vi "ME_acquire_4.vi"() -> ()   [LabVIEW 2015]
doc: "Use this template to build a producer/consumer design pattern. Use this template when you need to execute a process, such as data analysis, when a data source, such as a triggered acquisition, produces data at an uneven rate and you need to execute the process when the data becomes available."
uses:
  Mode.ctl
  oxford_driver/Oxford Drivers/BUSGEN.LLB/OxfordAddress.ctl
  <vilib>/Utility/file.llb/Write Delimited Spreadsheet (DBL).vi
  <vilib>/express/express arith-compare/Formula/XNode/ExpressFormulaBlockNode.xnode
  <vilib>/gmath/NI_Gmath.lvlib
panel:
  out "Actual B Field (T)":dbl
  out "Actual Temperature (K)":dbl
  out "Actual Current (pA)":dbl
  in  "Sweep Field":bool
  in  "Tab Control":T1(tab)
  out "P(T)":cluster{dbl[], dbl[]}(graph)
  out "I(T)":cluster{dbl[], dbl[]}(graph)
  in  "Set temperature (K)":dbl=4.5
  in  "Temp Ramping Rate (K/min)":dbl=10.0
  in  "Heater Range":enum16{"Off", "Low", "Medium", "High"}(ring)
  in  "Heater On/Off":bool
  out "I(B) /Averaged/":cluster{"B array":dbl[], dbl[]}[](graph)
  out "I(B) 3":cluster{dbl[], dbl[]}[](graph)
  in  "Go to Set":bool
  in  "Set Field (T)":dbl=0.3
  in  "Field To Zero":bool
  in  "Sweep Rate (T/min)":dbl=2.0 format="%.6f"
  in  "Min Field (T)":dbl
  in  "Max Field (T)":dbl
  out "Up/Down":bool
  in  "IV converter":refnum<visa-resource-name>="GPIB0::20::INSTR"
  in  "Magnetic Field":refnum<visa-resource-name>="GPIB0::21::INSTR"
  out "Time Lag":dbl=0.0500025749206543
  in  "Lake Shore":refnum<visa-resource-name>="GPIB0::11::INSTR"
  in  "Temp Refresh (s)":dbl=1.0
  in  "Sampling rate (Hz)":dbl=20.0
  in  "Gain (V/A)":dbl=1000.0
  in  "Sample area (mm^2)":dbl
  in  "dt (s)":dbl=0.05
  in  "Temp/Magnetic Field":bool
  out "Save":dbl[][](array[numeric])
  out "output array":dbl[][](array[numeric])
  out "index":i8
  out "Read?":bool
  out "Magnetic Field (T)":dbl[](array[numeric])
  out "Reset":bool
  out "Measured Current (pA)":dbl[](array[numeric])
  out "Elapsed Time (s)":dbl[](array[numeric])
  out "Start time":timestamp
  in  "Enum":T2
  out "B array":dbl[](array[numeric])
  in  "dB (T)":dbl=0.0001
  in  "Counter":i8
  out "L magnet (H)":dbl
  out "R magnet (mOhm)":dbl
  out "Actual Current (R0)":dbl
  out "Actual Field (T)":dbl
  out "Temperature array":dbl[](array[numeric])
  in  "New Measurement File":bool
  out "Measurement File":path
  out "refnum out":refnum<file>
  in  "Measuring":bool
  in  "Measure (Start/Pause)":bool
  in  "stop":bool
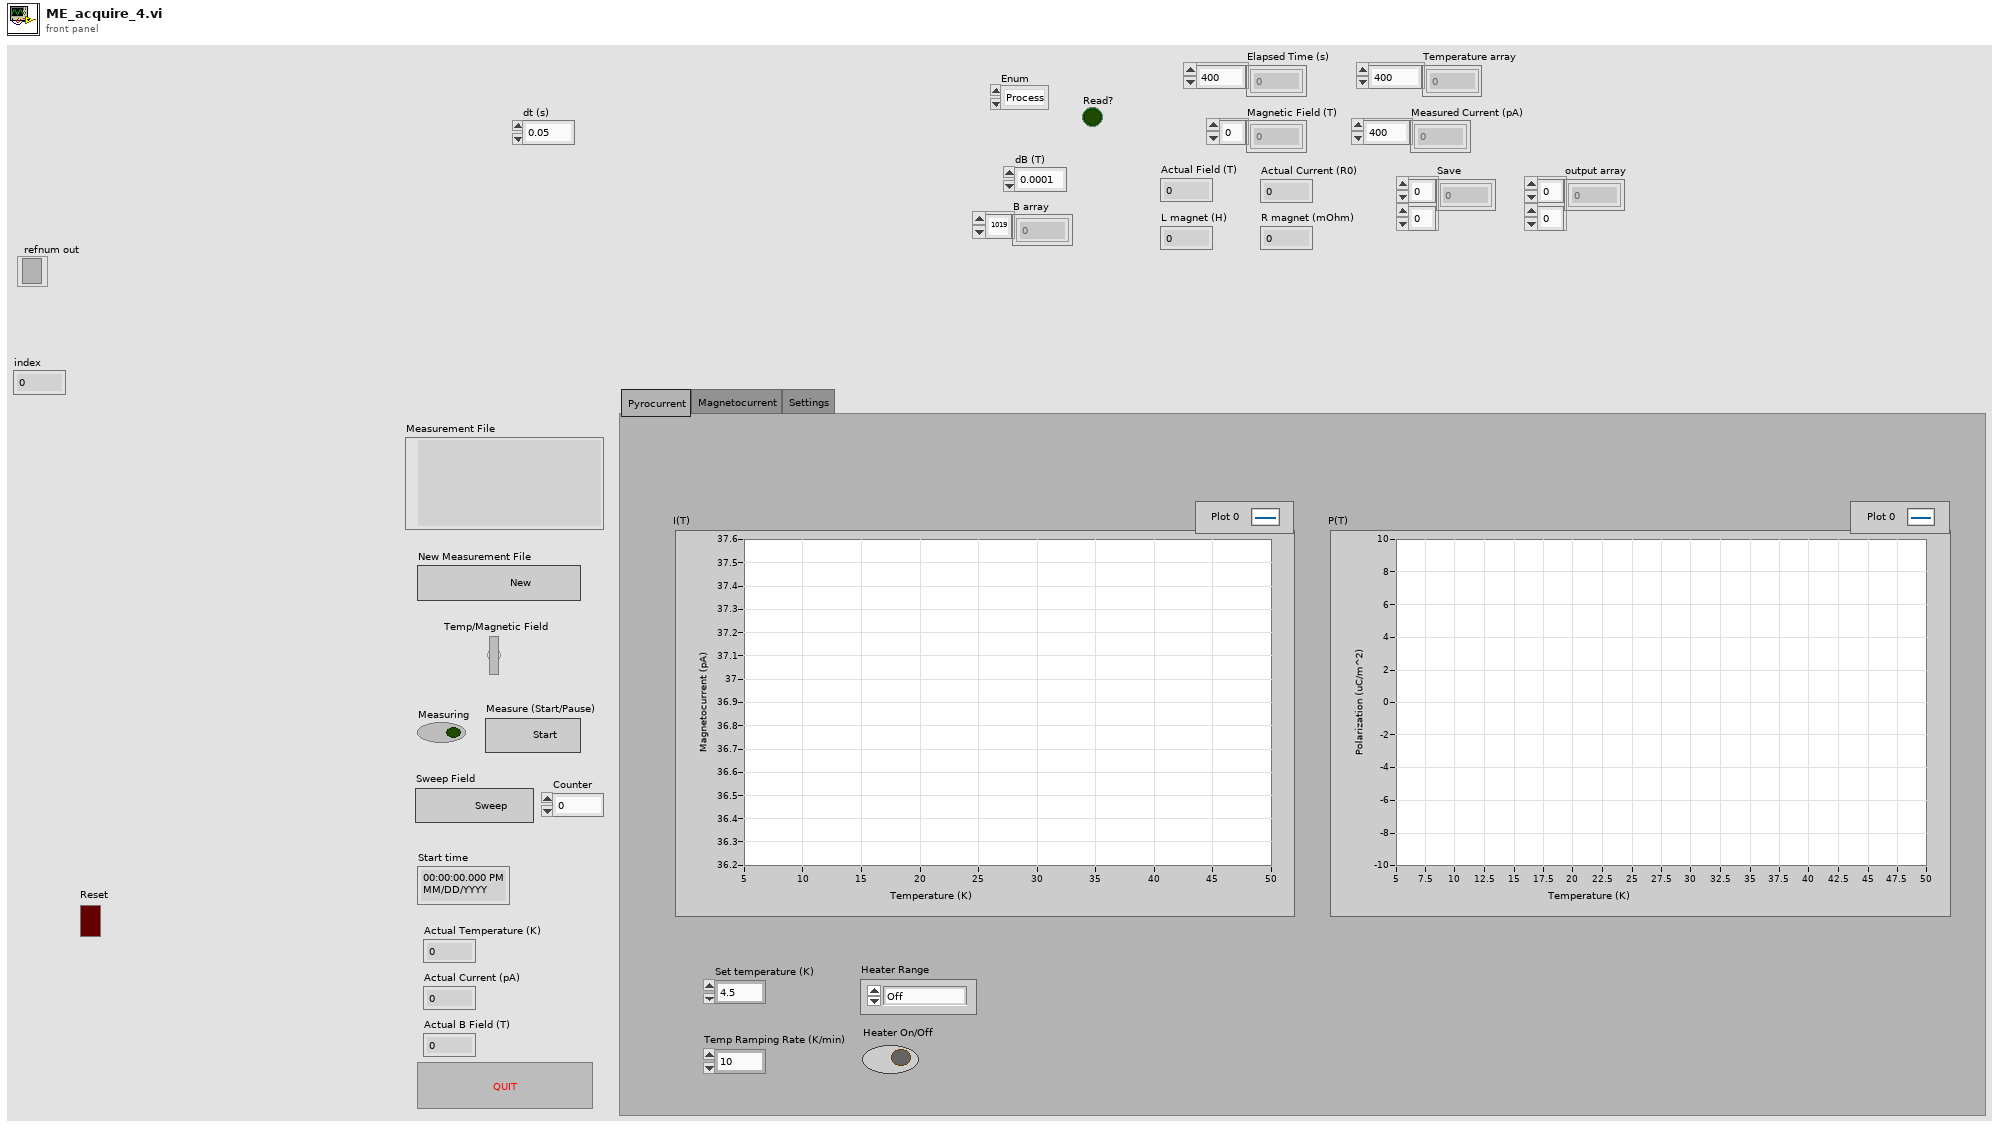
[diagram p1: front panel]
types:
  T1 = enum32{"Pyrocurrent", "Magnetocurrent", "Settings"}
  T2 = typedef "Mode.ctl" = enum16{"Process", "Plot", "Save", "Return"}
  T3 = enum16{"open", "replace", "create", "open or create", "replace or create", "replace or create with confirmation"}
  T4 = typedef "OxfordAddress.ctl" = cluster{"Com Port":i32, "ISOBUS Address":i32, "GPIB Address":i16, "Communication":enum16{"RS232", "ISOBUS", "GPIB", "Gateway"}}
  T5 = cluster{"seconds since 1Jan1904":timestamp, "read buffer":string, "read buffer":string}
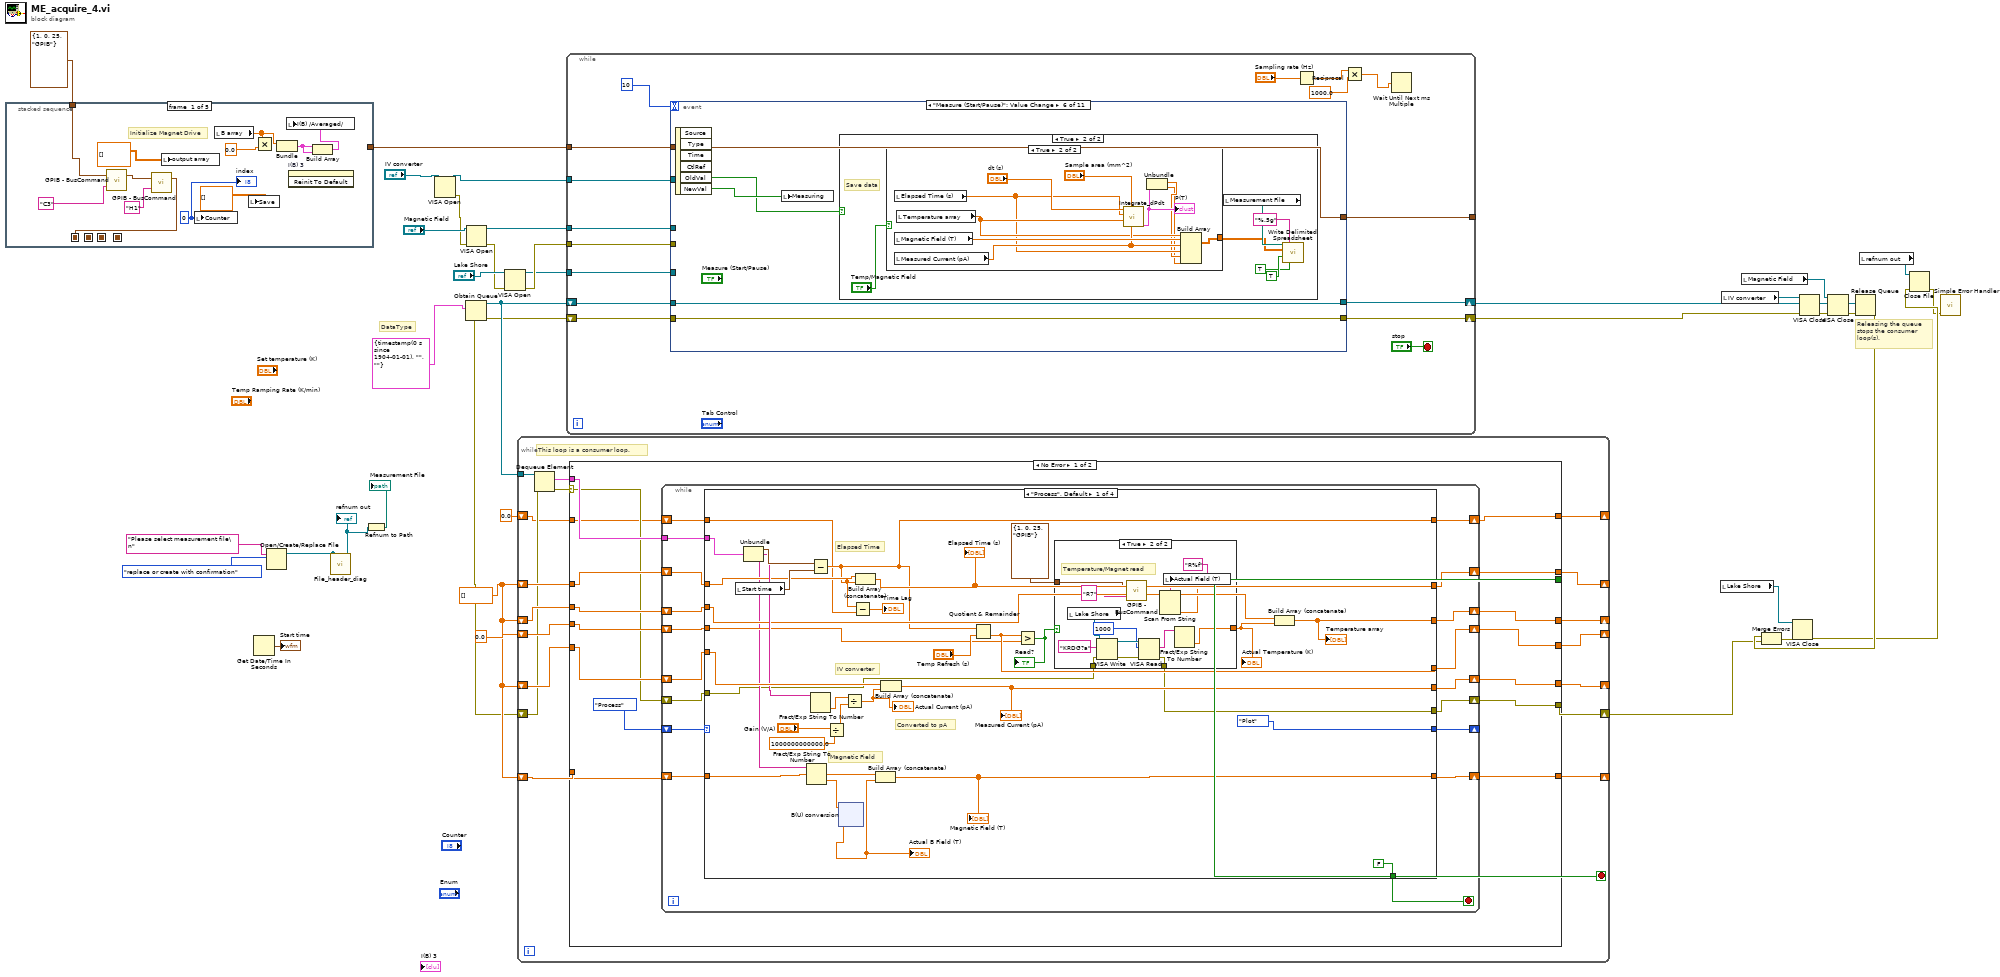
[diagram p0: block diagram]
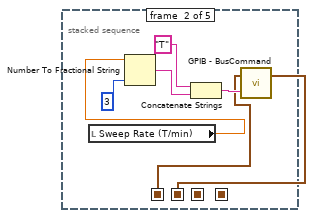
[diagram p2: hidden frame]
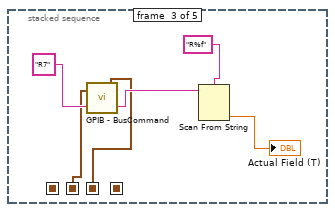
[diagram p3: hidden frame]
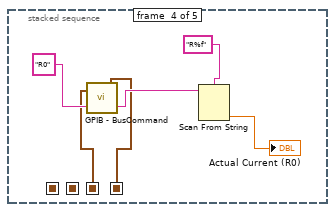
[diagram p4: hidden frame]
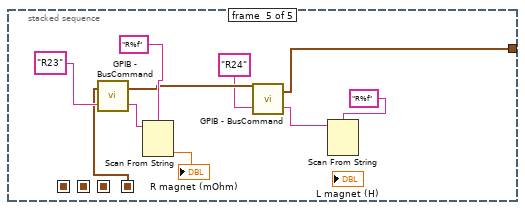
[diagram p5: hidden frame]
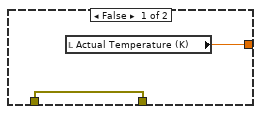
[diagram p6: hidden frame]
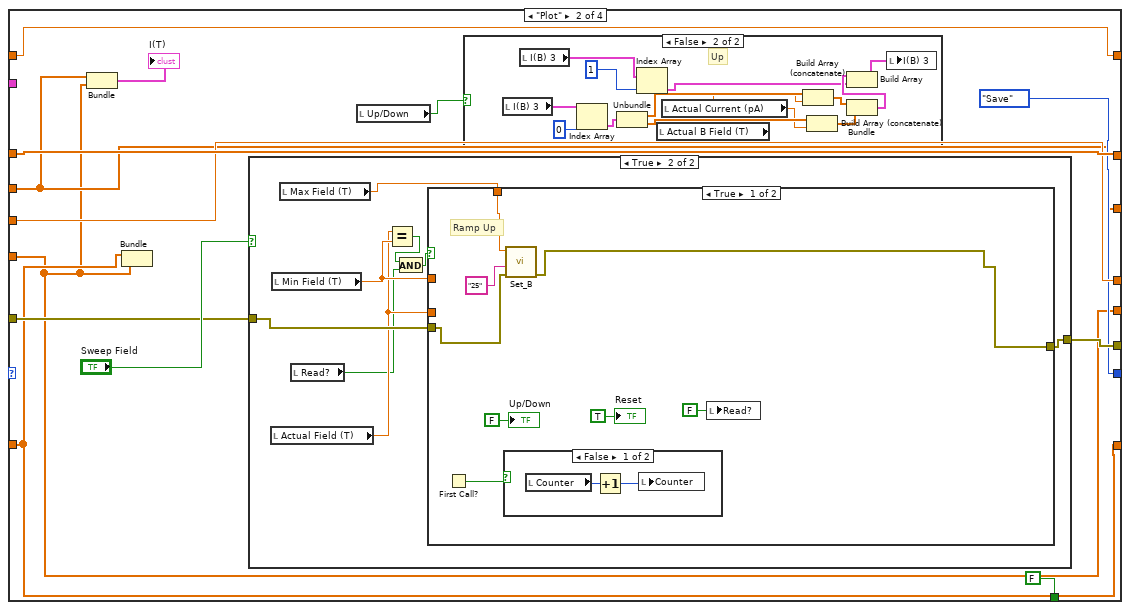
[diagram p7: hidden frame]
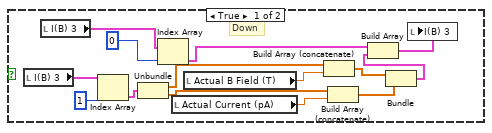
[diagram p8: hidden frame]
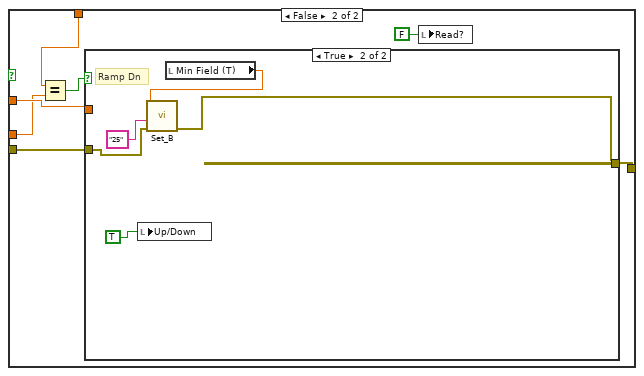
[diagram p11: hidden frame]
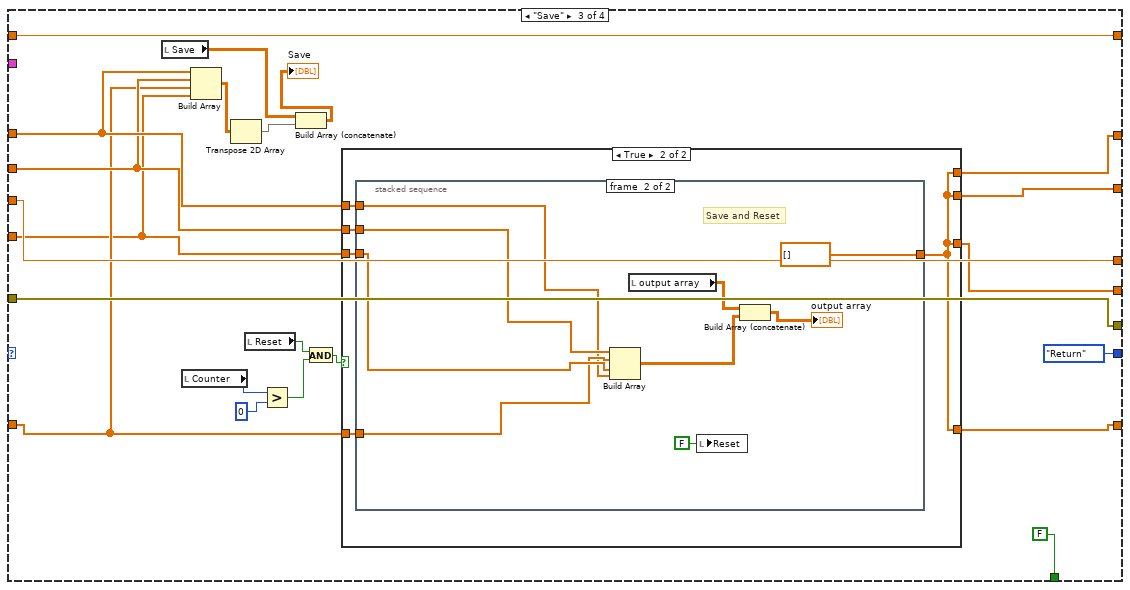
[diagram p13: hidden frame]
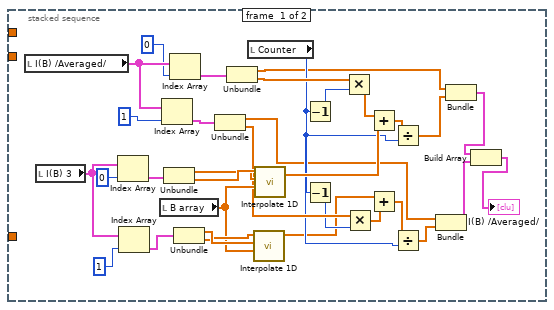
[diagram p15: hidden frame]
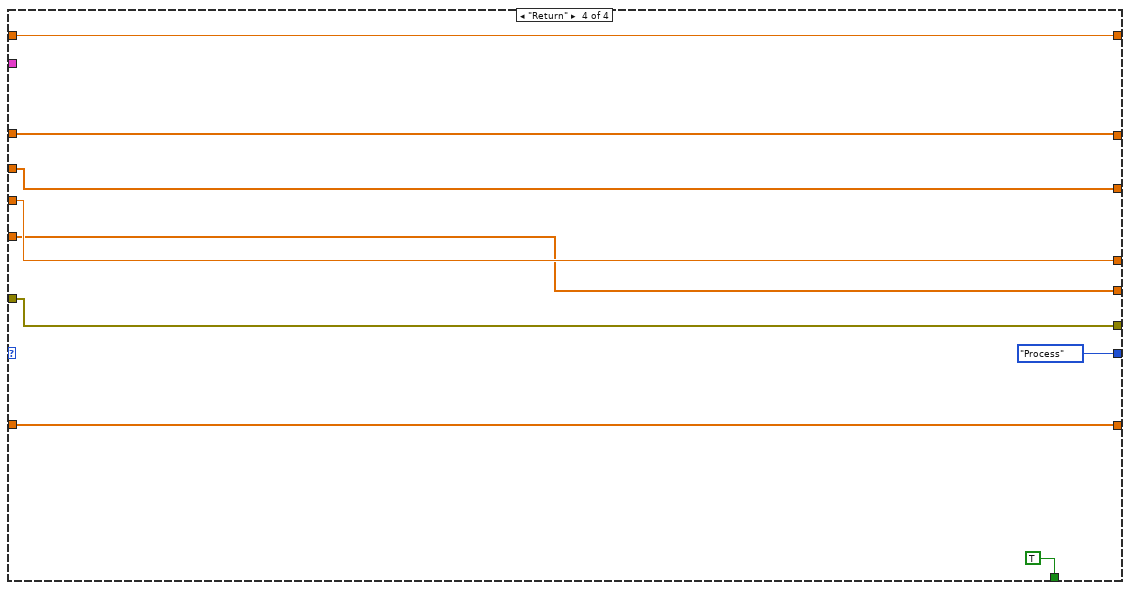
[diagram p16: hidden frame]
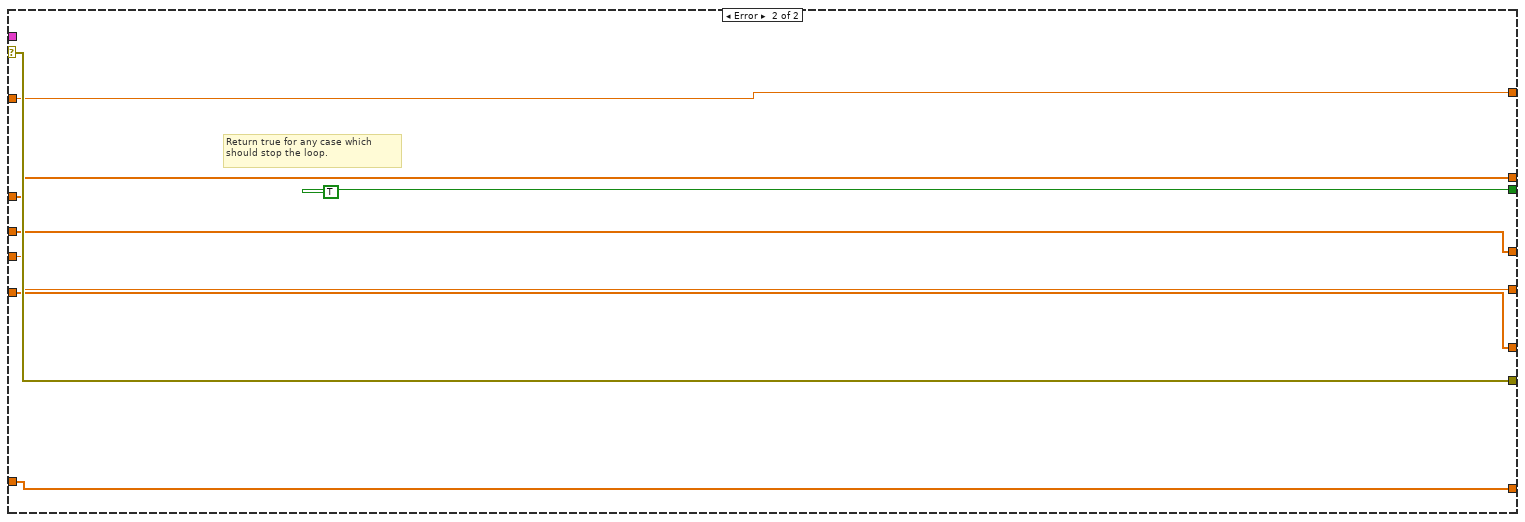
[diagram p17: hidden frame]
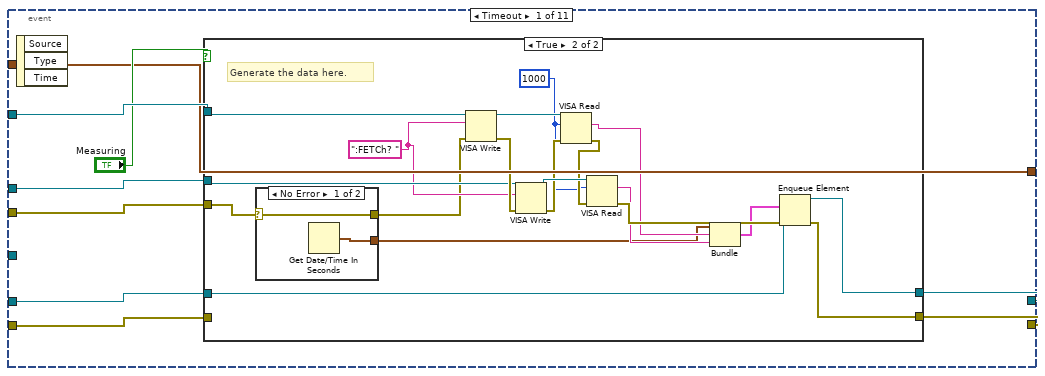
[diagram p18: hidden frame]
diagram:
  w5 = dbl[] []
  # "DataType"
  # "Releasing the queue stops the consumer loop(s)."
  n1 = stacked-sequence {
    seq-local: [w45 _ _ _ _] -> [_ w50 _ _ _]
    seq-local: [_ w49 _ _ _] -> [_ _ w57 _ _]
    seq-local: [_ _ w56 _ _] -> [_ _ _ w63 _]
    seq-local: [_ _ _ w62 _] -> [_ _ _ _ w73]
    tunnel: T4 {"Com Port"=1, "ISOBUS Address"=0, "GPIB Address"=25, "Communication"=enum."GPIB"} ("Address") -> [w47 _ _ _ _]
    tunnel: [_ _ _ _ w71] -> w14
    frame #0 {
      w43 = i8 0 ("Counter")
      # "Initialize Magnet Drive"
      n2 = call "GPIB - BusCommand.vi"("Command"="C3", "Address"=w47) -> ("Address(thru)"=w46:T4)  [unwired: 1 out]
      n3 = call "GPIB - BusCommand.vi"("Command"="H1", "Address"=w46) -> ("Address(thru)"=w45:T4)  [unwired: 1 out]
      n4 = local write "output array"(dbl[][] []) -> ()
      n5 = local write "Counter"(w43) -> ()
      n6 = local read "B array"() -> (w41:dbl[])
      n7 = local write "Save"(dbl[][] [] ("Save")) -> ()
      n8 = Multiply(x=w41, y=0.0) -> (x*y=w40:dbl[])
      n9 = Bundle("B array"=w41, w40) -> (w39:cluster{"B array":dbl[], dbl[]})  [unwired: 1 in]
      n10 = invoke on="I(B) 3" class="XYGraph (strict)" method="Reinit To Default"() -> ()  [unwired: 3 in, 3 out]
      n11 = Build Array(w39, w39) -> (w38:cluster{"B array":dbl[], dbl[]}[])
      n12 = local write "I(B) /Averaged/"(w38) -> ()
      "index" <- w43
    }
    frame #1 {
      n13 = local read "Sweep Rate (T/min)"() -> (w51:dbl)
      n14 = Number To Fractional String(number=w51, precision (6)=i16 3) -> (F-format string=w53:string)  [unwired: 2 in]
      n15 = Concatenate Strings("T" ("format string"), w53) -> (w52:string)
      n16 = call "GPIB - BusCommand.vi"("Command"=w52, "Address"=w50) -> ("Address(thru)"=w49:T4)  [unwired: 1 out]
    }
    frame #2 {
      n17 = call "GPIB - BusCommand.vi"("Command"="R7" ("format string"), "Address"=w57) -> ("Reply"=w61:string, "Address(thru)"=w56:T4)
      n18 = Scan From String(format string="R%f" ("remaining string"), input string=w61) -> (output 1=→"Actual Field (T)":dbl)  [unwired: 3 in, 3 out]
    }
    frame #3 {
      n19 = call "GPIB - BusCommand.vi"("Command"="R0" ("format string"), "Address"=w63) -> ("Reply"=w67:string, "Address(thru)"=w62:T4)
      n20 = Scan From String(format string="R%f" ("remaining string"), input string=w67) -> (output 1=→"Actual Current (R0)":dbl)  [unwired: 3 in, 3 out]
    }
    frame #4 {
      n21 = call "GPIB - BusCommand.vi"("Command"="R23" ("format string"), "Address"=w73) -> ("Reply"=w77:string, "Address(thru)"=w72:T4)
      n22 = Scan From String(format string="R%f" ("remaining string"), input string=w77) -> (output 1=→"R magnet (mOhm)":dbl)  [unwired: 3 in, 3 out]
      n23 = call "GPIB - BusCommand.vi"("Command"="R24" ("format string"), "Address"=w72) -> ("Reply"=w69:string, "Address(thru)"=w71:T4)
      n24 = Scan From String(format string="R%f" ("remaining string"), input string=w69) -> ()  [unwired: 4 in, 3 out]
    }
  }
  n25 = Get Date/Time In Seconds() -> (seconds since 1Jan1904=→"Start time":timestamp)
  n26 = Open/Create/Replace File(prompt="Please select measurement file\n", operation (0:open)=T3."replace or create with confirmation") -> (refnum out=w10:refnum<file>)  [unwired: 4 in, 2 out]
  "refnum out" <- w10
  n27 = call "File_header_diag.vi"("Byte Stream File in"=w10) -> ()  [unwired: 11 in]
  n28 = Refnum to Path(1:w10) -> (0:→"Measurement File":path)
  n29 = VISA Open(VISA resource name="IV converter") -> (VISA resource name=w30:refnum<visa-resource-name>, error out=w32:errorcluster)  [unwired: 4 in]
  n30 = Obtain Queue(element data type=T5 {"seconds since 1Jan1904"=timestamp(0 s since 1904-01-01), "read buffer"="", "read buffer"=""} ("output cluster")) -> (queue out=w35:refnum<queue>, error out=w3:errorcluster)  [unwired: 4 in, 1 out]
  n31 = VISA Open(error in (no error)=w32, VISA resource name="Magnetic Field") -> (VISA resource name=w29:refnum<visa-resource-name>, error out=w7:errorcluster)  [unwired: 3 in]
  n32 = VISA Open(error in (no error)=w7, VISA resource name="Lake Shore") -> (VISA resource name=w1:refnum<visa-resource-name>, error out=w6:errorcluster)  [unwired: 3 in]
  n33 = while {
    tunnel: w35 -> [w95]
    shift-right: [w90] -> _
    shift-left: w5 -> [w89]
    shift-right: [w88] -> _
    shift-left: w5 -> [w87]
    shift-right: [w86] -> _
    shift-left: w5 -> [w85]
    shift-right: [w84] -> _
    shift-left: 0.0 -> [w83]
    shift-right: [w82] -> _
    shift-left: w5 -> [w81]
    shift-right: [w91] -> w19
    shift-left: w3 -> [w80]
    shift-right: [w79] -> _
    shift-left: 0.0 -> [w78]
    stop <- w92 stop-if-true
    # "This loop is a consumer loop."
    n34 = Dequeue Element(queue=w95, error in (no error)=w80) -> (element=w93:T5, error out=w94:errorcluster)  [unwired: 1 in, 2 out]
    n35 = case shown="No Error" w94 {
      selector: w94 -> [w99 w348]
      tunnel: w93 -> [w110 _]
      tunnel: [_ TRUE] -> w92
      tunnel: [w98 w348] -> w91
      tunnel: [w109 w347] -> w90
      tunnel: w89 -> [w108 w347]
      tunnel: [w107 w344] -> w88
      tunnel: w87 -> [w106 w344]
      tunnel: [w105 w343] -> w86
      tunnel: w85 -> [w104 w343]
      tunnel: [w103 w345] -> w84
      tunnel: w83 -> [w102 w345]
      tunnel: [w101 w346] -> w82
      tunnel: w81 -> [w100 w346]
      tunnel: [w97 w342] -> w79
      tunnel: w78 -> [w96 w342]
      frame No Error {
        n36 = while {
          shift-right: [w117] -> _
          shift-left: Mode."Process" ("Enum") -> [w129]
          tunnel: w110 -> [w128]
          shift-right: [w127] -> w109
          shift-left: w108 -> [w126]
          shift-right: [w119] -> w101
          shift-left: w100 -> [w118]
          shift-right: [w121] -> w103
          shift-left: w102 -> [w120]
          shift-right: [w125] -> w107
          shift-left: w106 -> [w124]
          shift-right: [w115] -> w98
          shift-left: w99 -> [w116]
          shift-right: [w123] -> w105
          shift-left: w104 -> [w122]
          shift-right: [w113] -> w97
          shift-left: w96 -> [w112]
          stop <- w114 stop-if-true
          n37 = case shown="\"Process\", Default" w129 {
            tunnel: w128 -> [w160 _ _ _]
            tunnel: [w157 w196 w268 w340] -> w127
            tunnel: w126 -> [w148 w196 w267 w340]
            tunnel: [w156 w188 w270 w337] -> w125
            tunnel: w124 -> [w155 w188 w264 w337]
            tunnel: [w152 w192 w271 w334] -> w123
            tunnel: w122 -> [w151 w192 w265 w334]
            tunnel: [w147 w195 w279 w338] -> w121
            tunnel: w120 -> [w146 w195 w279 w338]
            tunnel: [w143 w189 w269 w339] -> w119
            tunnel: w118 -> [w144 w189 w266 w339]
            tunnel: [Mode."Plot" ("Enum") Mode."Save" ("Enum") Mode."Return" ("Enum") Mode."Process" ("Enum")] -> w117
            tunnel: w116 -> [w139 w198 w278 w336]
            tunnel: [w138 w197 w278 w336] -> w115
            tunnel: [FALSE FALSE FALSE TRUE] -> w114
            tunnel: [w135 w191 w277 w333] -> w113
            tunnel: w112 -> [w134 w191 w277 w333]
            frame "Process", Default {
              # "Converted to pA"
              # "Magnetic Field"
              # "IV converter"
              # "Elapsed Time"
              n38 = local read "Start time"() -> (w158:timestamp)
              n39 = Unbundle(w160) -> ("seconds since 1Jan1904"=w159:timestamp, "read buffer"=w153:string, "read buffer"=w140:string)
              n40 = Fract/Exp String To Number(string=w140) -> (number=w150:dbl)  [unwired: 3 in, 1 out]
              n41 = Subtract(x=w159, y=w158) -> (x-y=w135:dbl)
              n42 = Fract/Exp String To Number(string=w153) -> (number=w154:dbl)  [unwired: 3 in, 1 out]
              n43 = Divide(x="Gain (V/A)", y=1000000000000.0) -> (x/y=w132:dbl)
              n44 = xnode "B(U) conversion"("X1"=w150) -> ("Result"=w149:dbl)  [unwired: 1 in, 1 out]
              "Actual B Field (T)" <- w149
              n45 = Divide(x=w154, y=w132) -> (x/y=w133:dbl)
              "Actual Current (pA)" <- w133
              n46 = Subtract(x=w135, y=w134) -> (x-y=→"Time Lag":dbl)
              n47 = Build Array (concatenate)(w148, w135) -> (w157:dbl[])
              "Elapsed Time (s)" <- w157
              n48 = Build Array (concatenate)(w151, w149) -> (w152:dbl[])
              "Magnetic Field (T)" <- w152
              n49 = Build Array (concatenate)(w155, w133) -> (w156:dbl[])
              "Measured Current (pA)" <- w156
              n50 = Quotient & Remainder(x=w135, y="Temp Refresh (s)") -> (floor(x/y)=w147:dbl)  [unwired: 1 out]
              n51 = Greater?(x=w147, y=w146) -> (0:w145:bool)
              "Read?" <- w145
              n52 = case shown="True" w145 {
                tunnel: [w164 w172] -> w142
                tunnel: w139 -> [w163 w171]
                tunnel: [w163 w170] -> w138
                tunnel: T4 {"Com Port"=1, "ISOBUS Address"=0, "GPIB Address"=25, "Communication"=enum."GPIB"} ("Address") -> [_ w166]
                frame False {
                  n53 = local read "Actual Temperature (K)"() -> (w164:dbl)
                }
                frame True {
                  # "Temperature/Magnet read"
                  n54 = local read "Lake Shore"() -> (w173:refnum<visa-resource-name>)
                  n55 = VISA Write(VISA resource name=w173, write buffer="KRDG?a", error in (no error)=w171) -> (VISA resource name out=w177:refnum<visa-resource-name>, error out=w176:errorcluster)  [unwired: 1 out]
                  n56 = call "GPIB - BusCommand.vi"("Command"="R7" ("format string"), "Address"=w166) -> ("Reply"=w167:string)  [unwired: 1 out]
                  n57 = VISA Read(VISA resource name=w177, byte count=u32 1000, error in (no error)=w176) -> (read buffer=w174:string, error out=w170:errorcluster)  [unwired: 2 out]
                  n58 = Scan From String(format string="R%f" ("remaining string"), input string=w167) -> (output 1=w165:dbl)  [unwired: 3 in, 3 out]
                  n59 = local write "Actual Field (T)"(w165) -> ()
                  n60 = Fract/Exp String To Number(string=w174) -> (number=w172:dbl)  [unwired: 3 in, 1 out]
                }
              }
              "Actual Temperature (K)" <- w142
              n61 = Build Array (concatenate)(w144, w142) -> (w143:dbl[])
              "Temperature array" <- w143
            }
            frame "Plot" {
              n62 = Bundle(w189, w188) -> (→"I(T)":cluster{dbl[], dbl[]})  [unwired: 1 in]
              n63 = Bundle(w192, w188) -> ()  [unwired: 1 in, 1 out]
              n64 = case shown="True" "Sweep Field" {
                tunnel: [w228 w236] -> w197
                tunnel: w198 -> [w228 w233]
                frame False {
                }
                frame True {
                  n65 = local read "Actual Field (T)"() -> (w232:dbl)
                  n66 = local read "Min Field (T)"() -> (w234:dbl)
                  n67 = local read "Max Field (T)"() -> (w235:dbl)
                  n68 = local read "Read?"() -> (w229:bool)
                  n69 = Equal?(x=w232, y=w234) -> (x = y?=w231:bool)
                  n70 = And(x=w231, y=w229) -> (x .and. y?=w230:bool)
                  n71 = case shown="True" w230 {
                    tunnel: [w243 w253] -> w236
                    tunnel: w235 -> [w244 w252]
                    tunnel: w234 -> [_ w251]
                    tunnel: w232 -> [_ w249]
                    tunnel: w233 -> [w242 w248]
                    frame True {
                      # "Ramp Up"
                      n72 = First Call?() -> (First Call?: T/F=w237:bool)
                      n73 = case shown="False" w237 {
                        frame False {
                          n74 = local read "Counter"() -> (w245:i8)
                          n75 = Increment(x=w245) -> (x+1=w246:i8)
                          n76 = local write "Counter"(w246) -> ()
                        }
                        frame True {
                        }
                      }
                      n77 = call "Set_B.vi"("error in (no error)"=w242, "address string"="25", "Set Field (T)"=w244) -> ("error out"=w243:errorcluster)  [unwired: 8 in]
                      n78 = local write "Read?"(FALSE ("Read?")) -> ()
                      "Up/Down" <- FALSE ("Up/Down")
                      "Reset" <- TRUE ("Save")
                    }
                    frame False {
                      n79 = Equal?(x=w252, y=w249) -> (x = y?=w250:bool)
                      n80 = case shown="True" w250 {
                        tunnel: [w254 w256] -> w253
                        tunnel: w251 -> [_ _]
                        tunnel: w248 -> [w254 w257]
                        frame False {
                        }
                        frame True {
                          # "Ramp Dn"
                          n81 = local write "Up/Down"(TRUE ("Up/Down")) -> ()
                          n82 = local read "Min Field (T)"() -> (w255:dbl)
                          n83 = call "Set_B.vi"("error in (no error)"=w257, "address string"="25", "Set Field (T)"=w255) -> ("error out"=w256:errorcluster)  [unwired: 8 in]
                        }
                      }
                      n84 = local write "Read?"(FALSE ("Read?")) -> ()
                    }
                  }
                }
              }
              n85 = local read "Up/Down"() -> (w190:bool)
              n86 = case shown="False" w190 {
                frame True {
                  # "Down"
                  n87 = local read "I(B) 3"() -> (w209:cluster{dbl[], dbl[]}[])
                  n88 = local read "I(B) 3"() -> (w213:cluster{dbl[], dbl[]}[])
                  n89 = Index Array(array=w209, index=1) -> (element=w207:cluster{dbl[], dbl[]})
                  n90 = Unbundle(w207) -> (w206:dbl[], w205:dbl[])
                  n91 = Index Array(array=w213, index=i8 0 ("t")) -> (element=w210:cluster{dbl[], dbl[]})
                  n92 = local read "Actual Current (pA)"() -> (w202:dbl)
                  n93 = local read "Actual B Field (T)"() -> (w201:dbl)
                  n94 = Build Array (concatenate)(w206, w201) -> (w204:dbl[])
                  n95 = Build Array (concatenate)(w205, w202) -> (w203:dbl[])
                  n96 = Bundle(w204, w203) -> (w200:cluster{dbl[], dbl[]})  [unwired: 1 in]
                  n97 = Build Array(w210, w200) -> (w211:cluster{dbl[], dbl[]}[])
                  n98 = local write "I(B) 3"(w211) -> ()
                }
                frame False {
                  # "Up"
                  n99 = local read "I(B) 3"() -> (w225:cluster{dbl[], dbl[]}[])
                  n100 = local read "I(B) 3"() -> (w227:cluster{dbl[], dbl[]}[])
                  n101 = Index Array(array=w225, index=0) -> (element=w223:cluster{dbl[], dbl[]})
                  n102 = Unbundle(w223) -> (w222:dbl[], w221:dbl[])
                  n103 = Index Array(array=w227, index=i8 1 ("t")) -> (element=w215:cluster{dbl[], dbl[]})
                  n104 = local read "Actual B Field (T)"() -> (w217:dbl)
                  n105 = local read "Actual Current (pA)"() -> (w216:dbl)
                  n106 = Build Array (concatenate)(w222, w217) -> (w220:dbl[])
                  n107 = Build Array (concatenate)(w221, w216) -> (w219:dbl[])
                  n108 = Bundle(w220, w219) -> (w218:cluster{dbl[], dbl[]})  [unwired: 1 in]
                  n109 = Build Array(w218, w215) -> (w214:cluster{dbl[], dbl[]}[])
                  n110 = local write "I(B) 3"(w214) -> ()
                }
              }
            }
            frame "Save" {
              n111 = local read "Save"() -> (w260:dbl[][])
              n112 = local read "Counter"() -> (w276:i8)
              n113 = Build Array(w267, w266, w265, w264) -> (w263:dbl[][])
              n114 = Transpose 2D Array(2D array=w263) -> (transposed array=w262:dbl[][])
              n115 = local read "Reset"() -> (w273:bool)
              n116 = Greater?(x=w276, y=i8 0) -> (0:w272:bool)
              n117 = Build Array (concatenate)(w260, w262) -> (→"Save":dbl[][])
              n118 = And(x=w273, y=w272) -> (x .and. y?=w274:bool)
              n119 = case shown="True" w274 {
                tunnel: w265 -> [w285 w286]
                tunnel: [w285 w290] -> w271
                tunnel: w264 -> [w284 w287]
                tunnel: [w284 w290] -> w270
                tunnel: w266 -> [w283 w288]
                tunnel: [w283 w290] -> w269
                tunnel: w267 -> [w282 w289]
                tunnel: [w282 w290] -> w268
                frame False {
                }
                frame True {
                  n120 = stacked-sequence {
                    tunnel: [_ dbl[] []] -> w290
                    tunnel: w289 -> [_ w325]
                    tunnel: w288 -> [_ w330]
                    tunnel: w287 -> [_ w327]
                    tunnel: w286 -> [_ w326]
                    frame #0 {
                      n121 = local read "I(B) /Averaged/"() -> (w313:cluster{"B array":dbl[], dbl[]}[])
                      n122 = local read "I(B) 3"() -> (w320:cluster{dbl[], dbl[]}[])
                      n123 = Index Array(array=w320, index=0) -> (element=w319:cluster{dbl[], dbl[]})
                      n124 = Index Array(array=w320, index=1) -> (element=w321:cluster{dbl[], dbl[]})
                      n125 = local read "B array"() -> (w314:dbl[])
                      n126 = Index Array(array=w313, index=1) -> (element=w309:cluster{"B array":dbl[], dbl[]})
                      n127 = Unbundle(w319) -> (w317:dbl[], w318:dbl[])
                      n128 = Index Array(array=w313, index=0) -> (element=w310:cluster{"B array":dbl[], dbl[]})
                      n129 = Unbundle(w321) -> (w316:dbl[], w315:dbl[])
                      n130 = Unbundle(w309) -> ("B array"=w294:dbl[], w302:dbl[])
                      n131 = Unbundle(w310) -> ("B array"=w296:dbl[], w308:dbl[])
                      n132 = local read "Counter"() -> (w300:i8)
                      n133 = call <vilib>:"Interpolate 1D.vi"("xi"=w314, "X"=w316, "Y"=w315) -> ("yi"=w298:dbl[])  [unwired: 6 in, 2 out]
                      n134 = call <vilib>:"Interpolate 1D.vi"("xi"=w314, "X"=w317, "Y"=w318) -> ("yi"=w305:dbl[])  [unwired: 6 in, 2 out]
                      n135 = Decrement(x=w300) -> (x-1=w307:i8)
                      n136 = Decrement(x=w300) -> (x-1=w301:i8)
                      n137 = Multiply(x=w308, y=w307) -> (x*y=w306:dbl[])
                      n138 = Multiply(x=w302, y=w301) -> (x*y=w299:dbl[])
                      n139 = Add(x=w306, y=w305) -> (x+y=w304:dbl[])
                      n140 = Add(x=w298, y=w299) -> (x+y=w303:dbl[])
                      n141 = Divide(x=w304, y=w300) -> (x/y=w297:dbl[])
                      n142 = Divide(x=w303, y=w300) -> (x/y=w295:dbl[])
                      n143 = Bundle("B array"=w294, w295) -> (w292:cluster{"B array":dbl[], dbl[]})  [unwired: 1 in]
                      n144 = Bundle("B array"=w296, w297) -> (w293:cluster{"B array":dbl[], dbl[]})  [unwired: 1 in]
                      n145 = Build Array(w293, w292) -> (→"I(B) /Averaged/":cluster{"B array":dbl[], dbl[]}[])
                    }
                    frame #1 {
                      # "Save and Reset"
                      n146 = Build Array(w330, w326, w327, w325) -> (w324:dbl[][])
                      n147 = local read "output array"() -> (w329:dbl[][])
                      n148 = local write "Reset"(FALSE ("Save")) -> ()
                      n149 = Build Array (concatenate)(w329, w324) -> (→"output array":dbl[][])
                    }
                  }
                }
              }
            }
            frame "Return" {
            }
          }
        }
      }
      frame Error {
        # "Return true for any case which should stop the loop."
      }
    }
  }
  n150 = while {
    shift-right: [w361] -> w27
    shift-left: w3 -> [w362]
    shift-right: [w363] -> w34
    shift-left: w35 -> [w364]
    tunnel: w30 -> [w360]
    tunnel: w29 -> [w359]
    tunnel: w6 -> [w358]
    tunnel: [w352] -> _
    tunnel: w14 -> [w351]
    tunnel: w1 -> [w350]
    stop <- "stop" stop-if-true
    n151 = event shown="[5] \"Measure (Start/Pause)\": Value Change" {
      selector: _ -> [_ _ _ _ _ _ _ _ _ _ _]
      dyn-events: _ -> [_ _ _ _ _ _ _ _ _ _ _]
      timeout: 10 -> [_ _ _ _ _ _ _ _ _ _ _]
      tunnel: w364 -> [w374 w407 w417 w425 w436 w440 w464 w471 w487 w497 w508]
      tunnel: [w373 w407 w417 w425 w436 w440 w464 w471 w487 w497 w508] -> w363
      tunnel: w362 -> [w372 w406 w416 w426 w435 w444 w465 w473 w491 w501 w510]
      tunnel: [w371 w406 w416 w426 w437 w444 w465 w472 w490 w500 w509] -> w361
      tunnel: w360 -> [w370 _ _ _ _ _ _ _ _ _ _]
      tunnel: w359 -> [w369 _ _ _ _ _ _ _ _ _ _]
      tunnel: w358 -> [w368 _ _ _ _ _ _ _ _ _ _]
      tunnel: [w366 w405 w415 w424 w438 w441 w463 w470 w488 w498 _] -> w352
      tunnel: w351 -> [w366 w405 w418 w424 w438 w441 w463 w470 w488 w498 _]
      tunnel: w350 -> [_ _ _ _ _ _ _ w474 w489 w502 w507]
      event Timeout {
        n152 = event-data() -> ()  [unwired: 1 in, 3 out]
        n153 = case shown="True" "Measuring" {
          tunnel: w374 -> [w376 w395]
          tunnel: [w376 w394] -> w373
          tunnel: w372 -> [w375 _]
          tunnel: [w375 w393] -> w371
          tunnel: w370 -> [_ w386]
          tunnel: w369 -> [_ w385]
          tunnel: w368 -> [_ w380]
          frame False {
          }
          frame True {
            w383 = ":FETCh? " ("data")
            w387 = u32 1000 ("byte count")
            # "Generate the data here."
            n154 = case shown="No Error" w380 {
              selector: w380 -> [w397 w398]
              tunnel: [w397 w398] -> w379
              tunnel: [w396 _] -> w378
              frame No Error {
                n155 = Get Date/Time In Seconds() -> (seconds since 1Jan1904=w396:timestamp)
              }
              frame Error {
              }
            }
            n156 = VISA Write(VISA resource name=w386, write buffer=w383, error in (no error)=w379) -> (VISA resource name out=w392:refnum<visa-resource-name>, error out=w390:errorcluster)  [unwired: 1 out]
            n157 = VISA Write(VISA resource name=w385, write buffer=w383, error in (no error)=w390) -> (VISA resource name out=w391:refnum<visa-resource-name>, error out=w389:errorcluster)  [unwired: 1 out]
            n158 = VISA Read(VISA resource name=w392, byte count=w387, error in (no error)=w389) -> (read buffer=w381:string, error out=w388:errorcluster)  [unwired: 2 out]
            n159 = VISA Read(VISA resource name=w391, byte count=w387, error in (no error)=w388) -> (read buffer=w382:string, error out=w384:errorcluster)  [unwired: 2 out]
            n160 = Bundle("seconds since 1Jan1904"=w378, "read buffer"=w381, "read buffer"=w382) -> (w377:T5)  [unwired: 1 in]
            n161 = Enqueue Element(queue=w395, element=w377, error in (no error)=w384) -> (queue out=w394:refnum<queue>, error out=w393:errorcluster)  [unwired: 1 in, 1 out]
          }
        }
      }
      event "Max Field (T)": Value Change {
        n162 = event-data() -> ()  [unwired: 1 in, 6 out]
        n163 = Divide(x="Max Field (T)", y="dB (T)") -> (x/y=w402:dbl)
        n164 = Increment(x=w402) -> (x+1=w401:dbl)
        n165 = for {
          N: w401 -> [_]
          tunnel: "dB (T)" -> [w412]
          tunnel: [w409] -> w400 mode=indexing
          tunnel: "Min Field (T)" -> [w410]
          tunnel: [0.0] -> _ mode=indexing
          i -> [w414]
          n166 = Decrement(x=w414) -> (x-1=w413:i32)
          n167 = Multiply(x=w413, y=w412) -> (x*y=w411:dbl)
          n168 = Add(x=w411, y=w410) -> (x+y=w409:dbl)
        }
        "B array" <- w400
      }
      event "Sweep Rate (T/min)": Value Change {
        n169 = event-data() -> ("NewVal"=w422:dbl)  [unwired: 1 in, 5 out]
        n170 = Number To Fractional String(number=w422, precision (6)=i16 3) -> (F-format string=w420:string)  [unwired: 2 in]
        n171 = Concatenate Strings("T" ("format string"), w420) -> (w419:string)
        n172 = call "GPIB - BusCommand.vi"("Command"=w419, "Address"=w418) -> ("Address(thru)"=w415:T4)  [unwired: 1 out]
      }
      event "Field To Zero": Value Change {
        n173 = event-data() -> ()  [unwired: 1 in, 6 out]
        n174 = Two Button Dialog(message="Do you want to switch off the field?", 1:"No" ("F button name (\"Cancel\")"), 2:"Yes" ("T button name (\"OK\")")) -> (T button?=w430:bool)
        n175 = case shown="True" w430 {
          tunnel: w424 -> [_ w433]
          frame False {
          }
          frame True {
            n176 = local read "Sweep Rate (T/min)"() -> (w432:dbl)
            n177 = call "ips_switchHeaterOff.vi"("Instrument address"=w433, "Rate"=w432) -> ("B"=w431:dbl)
            n178 = local write "Actual Field (T)"(w431) -> ()
          }
        }
      }
      event "Go to Set": Value Change {
        n179 = event-data() -> ()  [unwired: 1 in, 6 out]
        n180 = call "Set_B.vi"("error in (no error)"=w435, "address string"="25", "Set Field (T)"="Set Field (T)") -> ("error out"=w437:errorcluster)  [unwired: 8 in]
      }
      event "Measure (Start/Pause)": Value Change {
        n181 = event-data() -> ("OldVal"=w442:bool, "NewVal"=w443:bool)  [unwired: 1 in, 4 out]
        n182 = local write "Measuring"(w443) -> ()
        n183 = case shown="True" w442 {
          frame False {
            n184 = local write "Temperature array"(dbl[] []) -> ()
          }
          frame True {
            # "Save data"
            n185 = case shown="True" "Temp/Magnetic Field" {
              tunnel: [w452 w461] -> w447
              frame False {
                n186 = local read "output array"() -> (w452:dbl[][])
              }
              frame True {
                n187 = local read "Magnetic Field (T)"() -> (w462:dbl[])
                n188 = local read "Measured Current (pA)"() -> (w460:dbl[])
                n189 = local read "Elapsed Time (s)"() -> (w457:dbl[])
                n190 = local read "Temperature array"() -> (w458:dbl[])
                n191 = call "Integrate_dPdt.vi"("Measured Current (pA)"=w460, "Sample area (mm^2)"="Sample area (mm^2)", "Temperature array"=w458, "Elapsed Time (s)"=w457, "dt (s)"="dt (s)") -> ("P(T)"=w456:cluster{"Temperature array":dbl[], dbl[]})  [unwired: 4 in, 2 out]
                "P(T)" <- w456
                n192 = Unbundle(w456) -> ("Temperature array"=w455:dbl[], w454:dbl[])
                n193 = Build Array(w458, w462, w460, w457, w455, w454) -> (w461:dbl[][])
              }
            }
            n194 = local read "Measurement File"() -> (w449:path)
            n195 = call-poly <vilib>:"Write Delimited Spreadsheet.vi"("file path (dialog if empty)"=w449, "format (%.3f)"="%.5g", "2D data"=w447, "append to file? (F)"=TRUE, "transpose? (F)"=TRUE) -> ()  [unwired: 9 in, 2 out]
          }
        }
      }
      event "New Measurement File": Value Change {
        n196 = event-data() -> ()  [unwired: 1 in, 6 out]
        n197 = Open/Create/Replace File(prompt="Please select measurement file\n", operation (0:open)=T3."replace or create with confirmation") -> (refnum out=w466:refnum<file>)  [unwired: 4 in, 2 out]
        n198 = local write "refnum out"(w466) -> ()
        n199 = Refnum to Path(1:w466) -> (0:w467:path)
        n200 = call "File_header_diag.vi"("Byte Stream File in"=w466) -> ()  [unwired: 11 in]
        n201 = local write "Measurement File"(w467) -> ()
      }
      event "Heater On/Off": Value Change {
        n202 = event-data() -> ()  [unwired: 1 in, 6 out]
        n203 = case shown="True" "Heater On/Off" {
          tunnel: w474 -> [w479 w485]
          tunnel: w473 -> [w477 w486]
          tunnel: [w476 w484] -> w472
          frame False {
            n204 = VISA Write(VISA resource name=w479, write buffer="RANGE,1,0", error in (no error)=w477) -> (error out=w476:errorcluster)  [unwired: 2 out]
          }
          frame True {
            n205 = Number To Decimal String(number="Heater Range") -> (decimal integer string=w482:string)  [unwired: 1 in]
            n206 = Concatenate Strings("RANGE,1," ("write buffer"), w482) -> (w480:string)
            n207 = VISA Write(VISA resource name=w485, write buffer=w480, error in (no error)=w486) -> (error out=w484:errorcluster)  [unwired: 2 out]
          }
        }
      }
      event "Set temperature (K)": Value Change {
        n208 = event-data() -> ()  [unwired: 1 in, 6 out]
        n209 = local read "Set temperature (K)"() -> (w492:dbl)
        n210 = Number To Fractional String(number=w492, precision (6)=i16 3) -> (F-format string=w495:string)  [unwired: 2 in]
        n211 = Concatenate Strings("SETP 1," ("write buffer"), w495) -> (w493:string)
        n212 = VISA Write(VISA resource name=w489, write buffer=w493, error in (no error)=w491) -> (error out=w490:errorcluster)  [unwired: 2 out]
      }
      event "Temp Ramping Rate (K/min)": Value Change {
        n213 = event-data() -> ()  [unwired: 1 in, 6 out]
        n214 = local read "Temp Ramping Rate (K/min)"() -> (w499:dbl)
        n215 = Number To Fractional String(number=w499, precision (6)=i16 1) -> (F-format string=w505:string)  [unwired: 2 in]
        n216 = Concatenate Strings("RAMP 1,1," ("string"), w505) -> (w504:string)
        n217 = VISA Write(VISA resource name=w502, write buffer=w504, error in (no error)=w501) -> (error out=w500:errorcluster)  [unwired: 2 out]
      }
      event "Heater Range": Value Change {
        n218 = event-data() -> ()  [unwired: 1 in, 6 out]
        n219 = local read "Heater On/Off"() -> (w511:bool)
        n220 = case shown="False" w511 {
          tunnel: w510 -> [w512 w517]
          tunnel: [w512 w516] -> w509
          tunnel: w507 -> [_ w515]
          frame False {
          }
          frame True {
            n221 = local read "Heater Range"() -> (w513:enum16{"Off", "Low", "Medium", "High"})
            n222 = Number To Decimal String(number=w513) -> (decimal integer string=w519:string)  [unwired: 1 in]
            n223 = Concatenate Strings("RANGE,1," ("write buffer"), w519) -> (w518:string)
            n224 = VISA Write(VISA resource name=w515, write buffer=w518, error in (no error)=w517) -> (error out=w516:errorcluster)  [unwired: 2 out]
          }
        }
      }
    }
    n225 = Reciprocal(x="Sampling rate (Hz)") -> (1/x=w356:dbl)
    n226 = Multiply(x=w356, y=1000.0) -> (x*y=w354:dbl)
    n227 = Wait Until Next ms Multiple(millisecond multiple=w354) -> ()  [unwired: 1 out]
  }
  n228 = local read "Lake Shore"() -> (w4:refnum<visa-resource-name>)
  n229 = local read "IV converter"() -> (w25:refnum<visa-resource-name>)
  n230 = local read "Magnetic Field"() -> (w24:refnum<visa-resource-name>)
  n231 = VISA Close(VISA resource name=w25, error in (no error)=w27) -> (error out=w28:errorcluster)
  n232 = VISA Close(VISA resource name=w24, error in (no error)=w28) -> (error out=w26:errorcluster)
  n233 = Release Queue(queue=w34, error in (no error)=w26) -> (error out=w20:errorcluster)  [unwired: 1 in, 2 out]
  n234 = Merge Errors(w20, w19) -> (w21:errorcluster)
  n235 = VISA Close(VISA resource name=w4, error in (no error)=w21) -> (error out=w18:errorcluster)
  n236 = local read "refnum out"() -> (w16:refnum<file>)
  n237 = Close File(refnum=w16, error in=w18) -> (error out=w17:errorcluster)  [unwired: 1 out]
  n238 = call <vilib>:"Simple Error Handler.vi"("error in (no error)"=w17) -> ()  [unwired: 4 in, 5 out]
